vi "__init__.vi"(6 "Wait Time (ms)":u32, 8 "error in":errorcluster, 9 "Driving Amplitude (V rms)":dbl, 10 "Lock-In Amplifier":refnum<class "Lock-In Amplifier.lvclass">, 11 "Function Generator":refnum<class "Function Generator.lvclass">) -> (0 "error out":errorcluster, 3 "Initialized Resonance Curve Measurement":refnum<class "Resonance Curve.lvclass">)   [LabVIEW 2020, in "Resonance Curve.lvclass"]
uses:
  Resonance Curve.lvclass
  Function Generator/Function Generator.lvclass
  Lock-In Amplifier/Lock-In Amplifier.lvclass
  Resonance Curve.lvclass/Resonance Curve.ctl
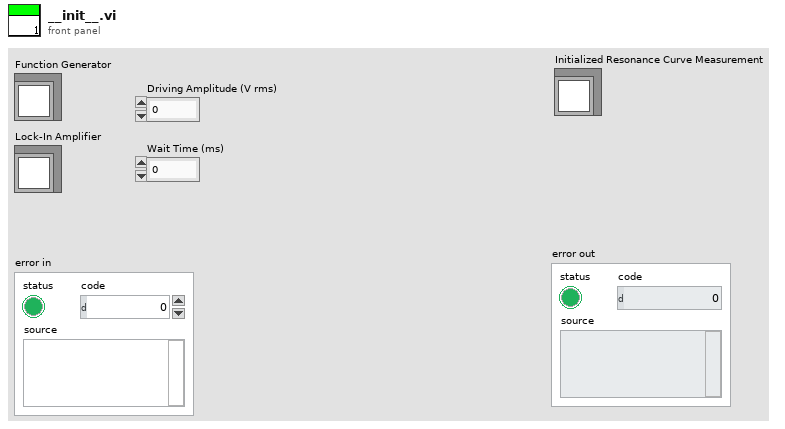
[diagram p1: front panel]
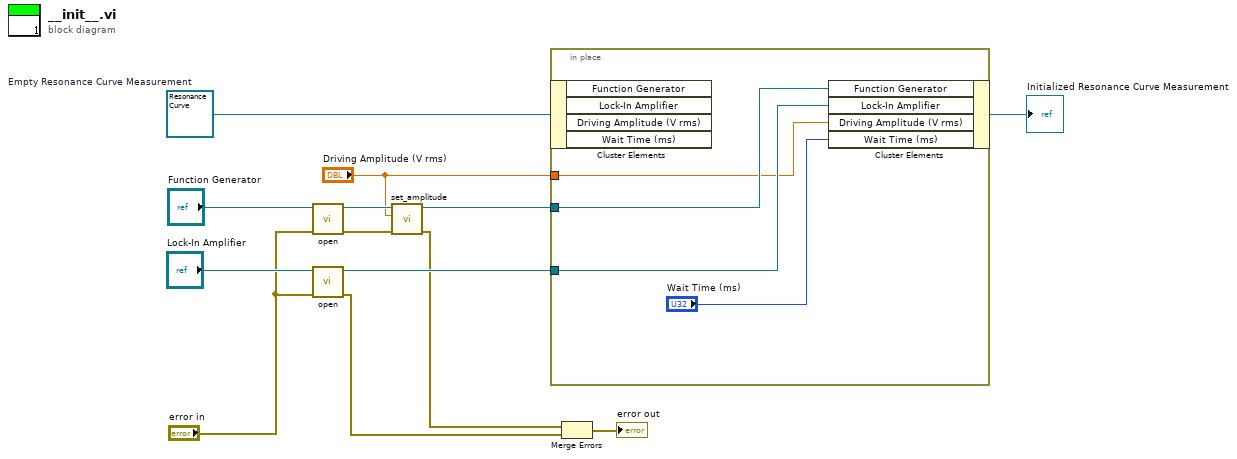
[diagram p0: block diagram]
diagram:
  w6 = refnum<class "Resonance Curve.lvclass"> refnum  # Empty Resonance Curve Measurement
  n1 = call-dynamic "open.vi"("error in (no error)"="error in", "Function Generator in"="Function Generator") -> ("error out"=w11:errorcluster, "Function Generator out"=w12:refnum<class "Function Generator.lvclass">)  [unwired: 8 in]
  n2 = call-dynamic "open.vi"("error in (no error)"="error in", "Instrument in"="Lock-In Amplifier") -> ("error out"=w2:errorcluster, "Instrument out"=w8:refnum<class "Lock-In Amplifier.lvclass">)  [unwired: 8 in]
  n3 = call-dynamic "set_amplitude.vi"("error in (no error)"=w11, "Amplitude"="Driving Amplitude (V rms)", "Function Generator in"=w12) -> ("error out"=w3:errorcluster, "Function Generator out"=w9:refnum<class "Function Generator.lvclass">)  [unwired: 7 in]
  n4 = in-place {
    in-place-border: w9 -> [w17]
    in-place-border: w8 -> [w16]
    in-place-border: "Driving Amplitude (V rms)" -> [w15]
    n5 = in-place-cluster #1(w6) -> ()  [unwired: 4 out]
    n6 = in-place-cluster #1("Function Generator"=w17, "Lock-In Amplifier"=w16, "Driving Amplitude (V rms)"=w15, "Wait Time (ms)"="Wait Time (ms)") -> (→"Initialized Resonance Curve Measurement":refnum<class "Resonance Curve.lvclass">)
  }
  n7 = Merge Errors(w3, w2) -> (→"error out":errorcluster)
